vi "Check Moving.vi"(8 "error in (no error)":errorcluster, 11 "VacuumLine in":refnum<class "VacuumLine.lvclass">) -> (0 "error out":errorcluster, 1 "Array of Checked-in?":bool[](array[boolean]), 2 "moving?":bool, 3 "VacuumLine out":refnum<class "VacuumLine.lvclass">)   [LabVIEW 2016, in "Hardware.lvlib" / "VacuumLine.lvlib" / "VacuumLine.lvclass"]
uses:
  <userlib>/Common Components/Hardware/Abstract System/VacuumLine/VacuumLine/VacuumLine.lvclass
  <userlib>/Common Components/Hardware/Abstract System/VacuumLine/VacuumLine/VacuumLine.lvclass/VacuumLine.ctl
  <userlib>/Common Components/Hardware/Motor/Motor/Motor.lvclass
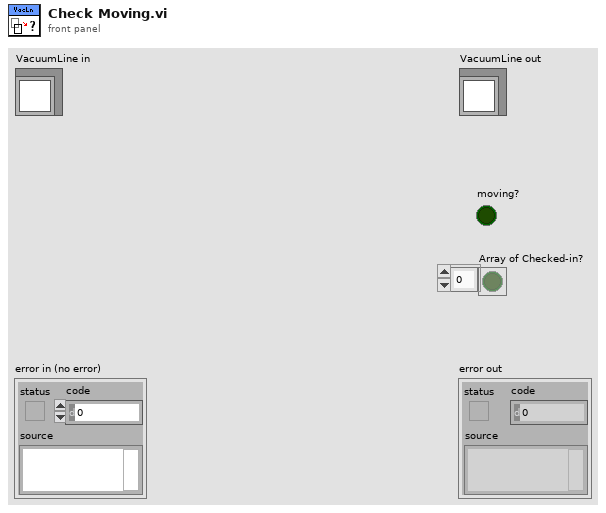
[diagram p1: front panel]
types:
  T1 = cluster{"valve":bool, "optical switch -":bool, "optical switch +":bool, "Valve Closed Status Alert":bool}[]
  T2 = typedef "Hardware.lvlib/VacuumLine.lvlib/VacuumLine.lvclass/Valve Complex.ctl" = cluster{"LogicIO Module":string, "Valve Open":T3, "Optical Switch -":T3, "Optical Switch +":T3, "Valve Closed Status Alert":cluster{"Pin#":u8, "Option":enum16{"Not Used", "Normally Closed"}}}
  T3 = typedef "Hardware.lvlib/VacuumLine.lvlib/VacuumLine.lvclass/Logic Cluster.ctl" = cluster{"Pin#":u8, "Location":dbl, "Tolerance":dbl}
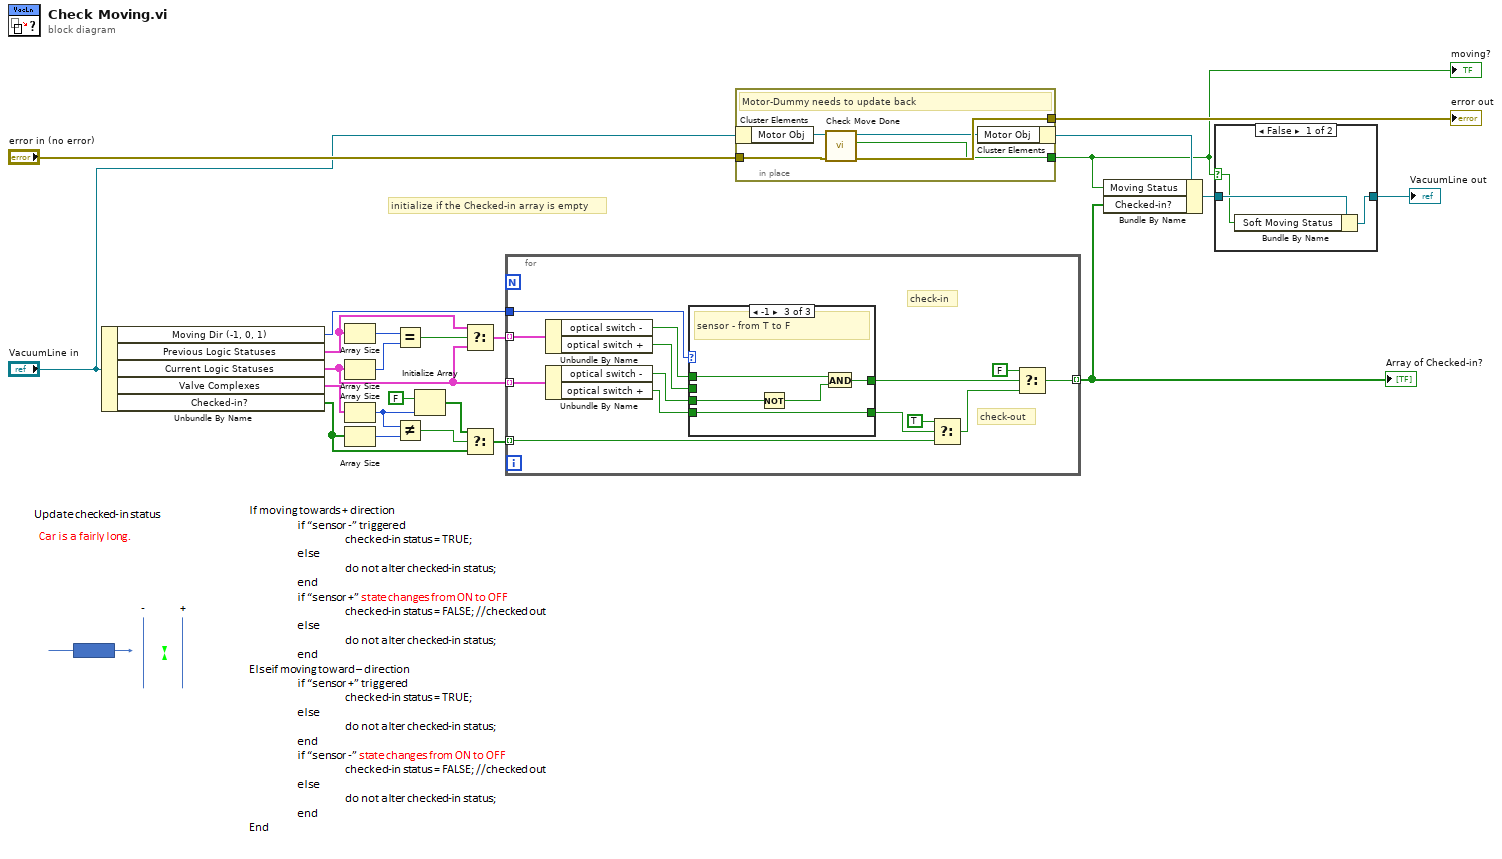
[diagram p0: block diagram]
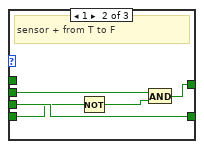
[diagram p4: hidden frame]
diagram:
  # "initialize if the Checked-in array is empty"
  n1 = Unbundle By Name("VacuumLine in") -> ("Moving Dir (-1, 0, 1)"=w19:i32, "Previous Logic Statuses"=w4:T1, "Current Logic Statuses"=w3:T1, "Valve Complexes"=w10:T2[], "Checked-in?"=w12:bool[])
  n2 = Array Size(array=w4) -> (size(s)=w6:i32)
  n3 = Array Size(array=w3) -> (size(s)=w7:i32)
  n4 = Array Size(array=w10) -> (size(s)=w9:i32)
  n5 = Array Size(array=w12) -> (size(s)=w16:i32)
  n6 = Equal?(x=w6, y=w7) -> (x = y?=w8:bool)
  n7 = Not Equal?(x=w9, y=w16) -> (x != y?=w15:bool)
  n8 = Initialize Array(FALSE, w9) -> (w13:bool[])
  n9 = Select(t=w4, s=w8, f=w3) -> (s? t:f=w5:T1)
  n10 = Select(t=w13, s=w15, f=w12) -> (s? t:f=w11:bool[])
  n11 = for {
    tunnel: w11 -> [w30] mode=indexing
    tunnel: [w27] -> w20 mode=indexing
    tunnel: w19 -> [w37]
    tunnel: w3 -> [w36] mode=indexing
    tunnel: w5 -> [w26] mode=indexing
    # "check-out"
    # "check-in"
    n12 = Unbundle By Name(w26) -> ("optical switch -"=w24:bool, "optical switch +"=w25:bool)
    n13 = Unbundle By Name(w36) -> ("optical switch -"=w35:bool, "optical switch +"=w34:bool)
    n14 = case shown="-1" w37 {
      tunnel: w35 -> [_ w42 w44]
      tunnel: w34 -> [_ w40 w47]
      tunnel: [_ w42 w47] -> w29
      tunnel: [_ w38 w43] -> w28
      tunnel: w25 -> [_ w41 _]
      tunnel: w24 -> [_ _ w45]
      frame 0, Default {
      }
      frame 1 {
        # "sensor + from T to F"
        n15 = Not(x=w40) -> (.not. x?=w39:bool)
        n16 = And(x=w41, y=w39) -> (x .and. y?=w38:bool)
      }
      frame -1 {
        # "sensor - from T to F"
        n17 = Not(x=w44) -> (.not. x?=w46:bool)
        n18 = And(x=w45, y=w46) -> (x .and. y?=w43:bool)
      }
    }
    n19 = Select(t=TRUE, s=w29, f=w30) -> (s? t:f=w32:bool)
    n20 = Select(t=FALSE, s=w28, f=w32) -> (s? t:f=w27:bool)
  }
  "Array of Checked-in?" <- w20
  n21 = in-place {
    in-place-border: "error in (no error)" -> [w52]
    in-place-border: [w51] -> w22
    in-place-border: [w50] -> w1
    # "Motor-Dummy needs to update back"
    n22 = in-place-cluster #1("VacuumLine in") -> ("Motor Obj"=w49:refnum<class "Motor.lvclass">)
    n23 = call-dynamic "Check Move Done.vi"("error in (no error)"=w52, "Motor in"=w49) -> ("error out"=w51:errorcluster, "moving?"=w50:bool, "Motor out"=w48:refnum<class "Motor.lvclass">)  [unwired: 7 in]
    n24 = in-place-cluster #1("Motor Obj"=w48) -> (w17:refnum<class "VacuumLine.lvclass">)
  }
  "error out" <- w22
  "moving?" <- w1
  n25 = Bundle By Name(cluster=w17, "Moving Status"=w1, "Checked-in?"=w20) -> (w21:refnum<class "VacuumLine.lvclass">)
  n26 = case shown="False" w1 {
    selector: w1 -> [w53 _]
    tunnel: w21 -> [w55 w56]
    tunnel: [w54 w56] -> w2
    frame False {
      n27 = Bundle By Name(cluster=w55, "Soft Moving Status"=w53) -> (w54:refnum<class "VacuumLine.lvclass">)
    }
    frame True {
    }
  }
  "VacuumLine out" <- w2
